vi "TPNT_GetLogPath.vi"(11 "logpath in":path) -> (3 "logpath out":path)   [LabVIEW 2016]
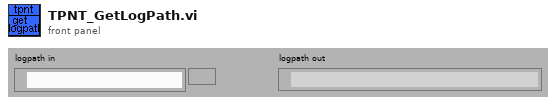
[diagram p1: front panel]
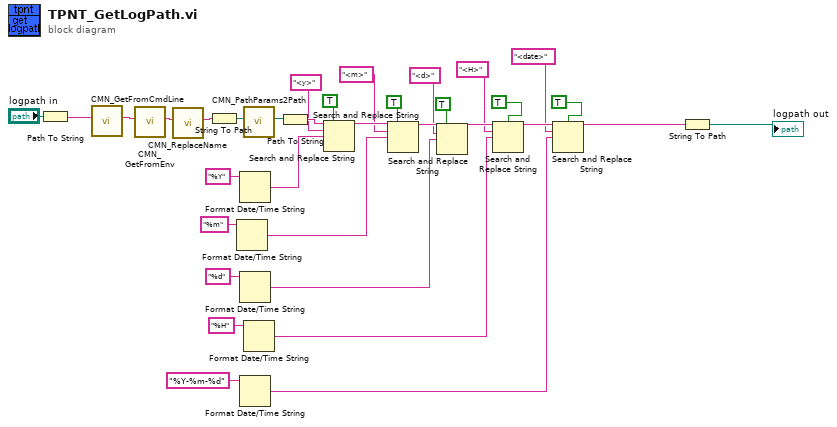
[diagram p0: block diagram]
diagram:
  n1 = Path To String(path="logpath in") -> (string=w32:string)
  n2 = call "CMN_GetFromCmdLine.vi"("str in"=w32) -> ("str out"=w34:string)  [unwired: 10 out]
  n3 = call "CMN_GetFromEnv.vi"("str in"=w34) -> ("str out"=w31:string)  [unwired: 10 out]
  n4 = call "CMN_ReplaceName.vi"("name in"=w31) -> ("name out"=w30:string)  [unwired: 1 in, 9 out]
  n5 = String To Path(string=w30) -> (path=w29:path)
  n6 = Format Date/Time String(time format string (%c)="%m") -> (date/time string=w17:string)  [unwired: 2 out]
  n7 = Format Date/Time String(time format string (%c)="%Y") -> (date/time string=w23:string)  [unwired: 2 out]
  n8 = Format Date/Time String(time format string (%c)="%d") -> (date/time string=w14:string)  [unwired: 2 out]
  n9 = Format Date/Time String(time format string (%c)="%Y-%m-%d") -> (date/time string=w1:string)  [unwired: 2 out]
  n10 = call "CMN_PathParams2Path.vi"("Path In"=w29) -> ("Path out"=w28:path)  [unwired: 2 in, 8 out]
  n11 = Format Date/Time String(time format string (%c)="%H") -> (date/time string=w8:string)  [unwired: 2 out]
  n12 = Path To String(path=w28) -> (string=w27:string)
  n13 = Search and Replace String(replace all?=TRUE ("replace all? (F)"), input string=w27, search string="<y>", replace string=w23) -> (result string=w21:string)  [unwired: 1 in, 6 out]
  n14 = Search and Replace String(replace all?=TRUE ("replace all? (F)"), input string=w21, search string="<m>", replace string=w17) -> (result string=w15:string)  [unwired: 1 in, 6 out]
  n15 = Search and Replace String(replace all?=TRUE ("replace all? (F)"), input string=w15, search string="<d>", replace string=w14) -> (result string=w11:string)  [unwired: 1 in, 6 out]
  n16 = Search and Replace String(case sensitive?=TRUE ("replace all? (F)"), input string=w11, search string="<H>", replace string=w8) -> (result string=w5:string)  [unwired: 1 in, 6 out]
  n17 = Search and Replace String(case sensitive?=TRUE ("replace all? (F)"), input string=w5, search string="<date>", replace string=w1) -> (result string=w4:string)  [unwired: 1 in, 6 out]
  n18 = String To Path(string=w4) -> (path=→"logpath out":path)
